vi "SCP Upload File.vi"(8 "Error In":errorcluster, 9 "Target Directory":string="/home/debian/", 10 "Local File":path, 11 "SCP Session":refnum<k24>) -> (0 "Error Out":errorcluster, 3 "SCP Session":refnum<k24>)   [LabVIEW 2020, in "LMH-LINX.lvlib"]
uses:
  LMH-LINX.lvlib
  c:/p4/penguin/lvaddon/MakerHub/LINX/trunk/20.1/objects/MakerHub_LINX/win32U/i386/msvc90/release/LabVIEW/vi.lib/MakerHub/LINX/Resources/Renci.SshNet.dll
  Resources/Renci.SshNet.dll
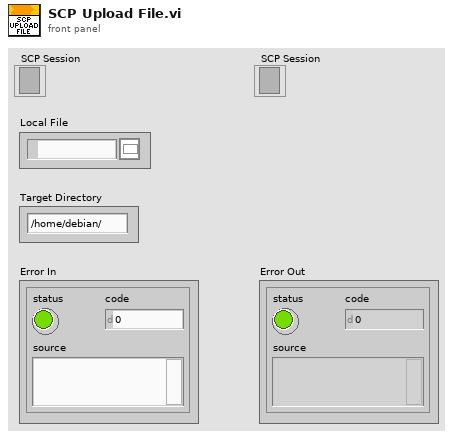
[diagram p1: front panel]
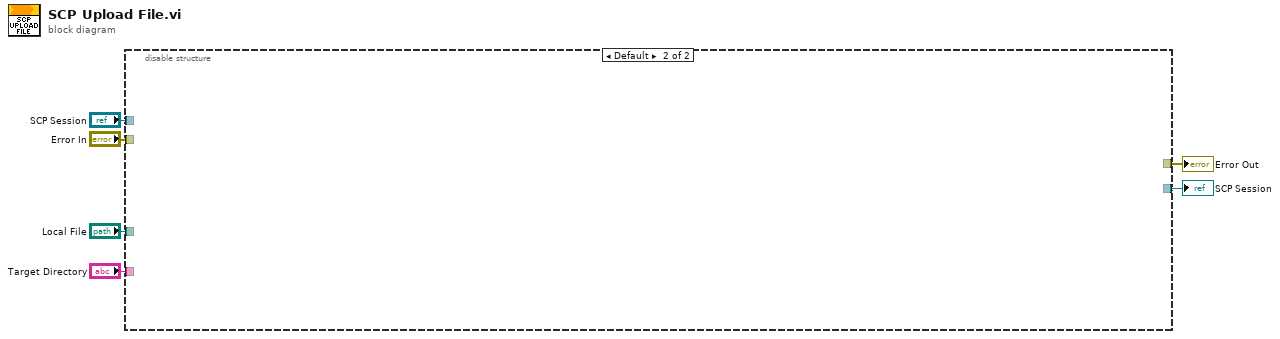
[diagram p0: block diagram]
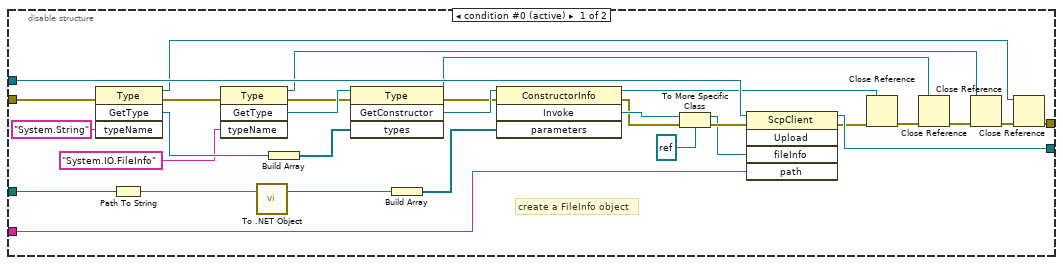
[diagram p2: hidden frame]
diagram:
  n1 = disable-structure shown="Default" {
    disable-tunnel: "Local File" -> [w36 _]
    disable-tunnel: "Target Directory" -> [w35 _]
    disable-tunnel: "Error In" -> [w33 _]
    disable-tunnel: [w21 _] -> w3
    disable-tunnel: "SCP Session" -> [w20 _]
    disable-tunnel: [w7 _] -> w1
    frame condition #0 (active) {
      # "create a FileInfo object"
      n2 = invoke class="Type" method="GetType"(error in=w33, "typeName"="System.String") -> (reference out=w8:refnum<k24>, error out=w19:errorcluster, "GetType"=w25:refnum<k24>)  [unwired: 2 in, 1 out]
      n3 = Path To String(path=w36) -> (string=w37:string)
      n4 = invoke class="Type" method="GetType"(error in=w19, "typeName"="System.IO.FileInfo") -> (reference out=w10:refnum<k24>, error out=w18:errorcluster, "GetType"=w23:refnum<k24>)  [unwired: 2 in, 1 out]
      n5 = call <vilib>:"To .NET Object.vi"("anything"=w37) -> (".NET object"=w28:refnum<k24>)  [unwired: 1 in, 1 out]
      n6 = Build Array(w25) -> (w27:refnum<k24>[])
      n7 = invoke class="Type" method="GetConstructor"(reference=w23, error in=w18, "types"=w27) -> (reference out=w11:refnum<k24>, error out=w17:errorcluster, "GetConstructor"=w26:refnum<k24>)  [unwired: 1 in, 1 out]
      n8 = Build Array(w28) -> (w29:refnum<k24>[])
      n9 = invoke class="ConstructorInfo" method="Invoke"(reference=w26, error in=w17, "parameters"=w29) -> (reference out=w14:refnum<k24>, error out=w16:errorcluster, "Invoke"=w31:refnum<k24>)  [unwired: 1 in, 1 out]
      n10 = To More Specific Class(target class=refnum<k24> refnum ("fileInfo"), reference=w31, error in=w16) -> (specific class reference=w32:refnum<k24>, error out=w34:errorcluster)
      n11 = invoke class="ScpClient" method="Upload"(reference=w20, error in=w34, "fileInfo"=w32, "path"=w35) -> (reference out=w21:refnum<k24>, error out=w15:errorcluster)  [unwired: 1 in, 3 out]
      n12 = Close Reference(reference=w14, error in (no error)=w15) -> (error out=w13:errorcluster)
      n13 = Close Reference(reference=w11, error in (no error)=w13) -> (error out=w12:errorcluster)
      n14 = Close Reference(reference=w10, error in (no error)=w12) -> (error out=w9:errorcluster)
      n15 = Close Reference(reference=w8, error in (no error)=w9) -> (error out=w7:errorcluster)
    }
    frame condition #1 {
    }
  }
  "Error Out" <- w1
  "SCP Session" <- w3
